vi "pick_and_place_sorting_weights_project.vi"() -> ()   [LabVIEW 2023]
uses:
  <vilib>/MakerHub/LINX/Public/Peripherals/Digital/Digital Write 1 Chan.vi
  <vilib>/MakerHub/LINX/Public/Peripherals/Digital/Digital Write N Chans.vi
  <vilib>/MakerHub/LINX/Private/Local IO/LinxDigitalWrite.vi
  <vilib>/MakerHub/LINX/Public/Utilities/Check Channel.vi
  <vilib>/MakerHub/LINX/Public/Utilities/Open Serial.vi
  <vilib>/MakerHub/LINX/Public/Sensors/Motion/Servo/Servo Open N Channels.vi
  <vilib>/Instr/_visa.llb/VISA Configure Serial Port (Instr).vi
  <vilib>/MakerHub/LINX/Private/Utilties/Generate Error.vi
  <vilib>/MakerHub/LINX/Public/Sensors/Motion/Servo/Servo Set Pulse Width N Channels.vi
  <vilib>/MakerHub/LINX/Public/Sensors/Motion/Servo/Servo Close N Channels.vi
  <vilib>/MakerHub/LINX/LMH-LINX.lvlib
  <vilib>/MakerHub/LINX/Public/Sensors/Motion/Servo/Servo.lvlib
panel:
  in  "load cell arduino serial port":refnum<visa-resource-name>="N/A"
  out "TO POS":i32[](array[numeric])
  out "FROM POS":i32[](array[numeric])
  out "CURRENT\nBOX POS":i32
  in  "main arduino serial port":refnum<visa-resource-name>="N/A"
  in  "lift servo\nchannel":u8 max=50 step=1
  in  "rotate servo\nchannel":u8 max=50 step=1
  in  "magnet\nchannel":u8 max=50 step=1
  in  "AUTO SORTING WEIGHTS":bool
  out "CONTROL MODE":bool
  in  "STOP PROGRAM":bool
  in  "BOXES POSITIONS":bool[](array[boolean])
  in  "LIFT":u32(slide) max=100 step=5 scale=0.0..100.0
  in  "MAGNET":bool caption="Boolean 2"
  out "BOXES WEIGHTS MEASUREMENTS":dbl[](array[numeric])
  out "CURRENT WEIGHT":dbl format="%#.1p"
  in  "ROTATE":u32(knob) caption="Up Button" max=260 step=5
  # "Pick and Place - Sorting Weights"
  # "Robotic arm control"
  # "Scale / weights control"
  # "1               2               3               4"
  # "o"
  # "%"
  # "gr"
  # "Initially, give the correct serial communication USB ports for the two arduinos and the right pins numbers to the servo, magnet and load cell channels, and then run the program. You can control the robotic arm manually (the joints' servomotors and the electromagent) using the controls of the \"Robotic arm control\" section. To start the \"auto sorting weights\" process, first you have to mark the positions of the boxes in the \"Scale / weights control\" section, before pressing the appropriate button."
  # "Boxes positions:\n1 -> 50 degrees\n2 -> 80 degrees\n3 -> 110 degrees\n4 -> 140 degrees\nScale position:\n5 -> 3 degrees"
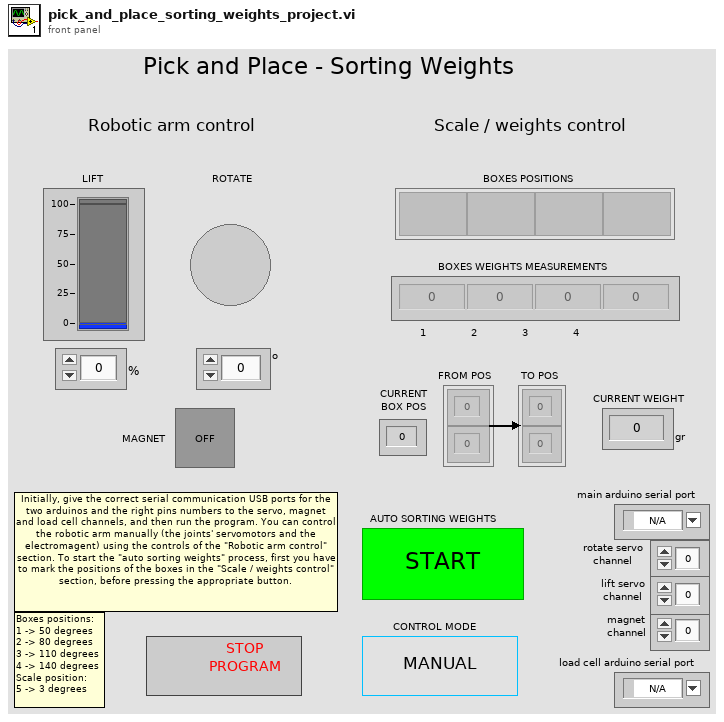
[diagram p1: front panel]
types:
  T1 = typedef "LMH-LINX.lvlib/LINX Ref.ctl" = cluster{"IO":T2, "Interface":T3, "LINX Device Config":T4}
  T2 = typedef "LMH-LINX.lvlib/Platform.ctl" = enum16{"Remote", "Local"}
  T3 = typedef "LMH-LINX.lvlib/Interface.ctl" = enum16{"Serial", "TCP"}
  T4 = typedef "LMH-LINX.lvlib/Device.lvlib/LINX Device Config.ctl" = cluster{"Interface":T3, "COM Port":refnum<visa-resource-name>, "TCP Configuration":T5, "Device Family":u8, "Device ID":u8, "Device Name":string, "TCP Ref":refnum<k5>, "Channels":T6}
  T5 = typedef "LMH-LINX.lvlib/Device.lvlib/TCP Config.ctl" = cluster{"IP Address":string, "Port":u16}
  T6 = typedef "LMH-LINX.lvlib/Channels.ctl" = cluster{"DI":u8[], "DO":u8[], "AI":u8[], "AO":u8[], "PWM":u8[], "QE":u8[], "UART":u8[], "I2C 2":u8[], "SPI":u8[], "CAN":u8[], "Servo":u8[], "AI Ref (V)":dbl, "AI Resolution (Bits)":u8, "AO Ref (V)":dbl, "AO Resolution (Bits)":u8}
  T7 = enum8{"Enabled", "Disabled", "Disabled and Grayed Out"}
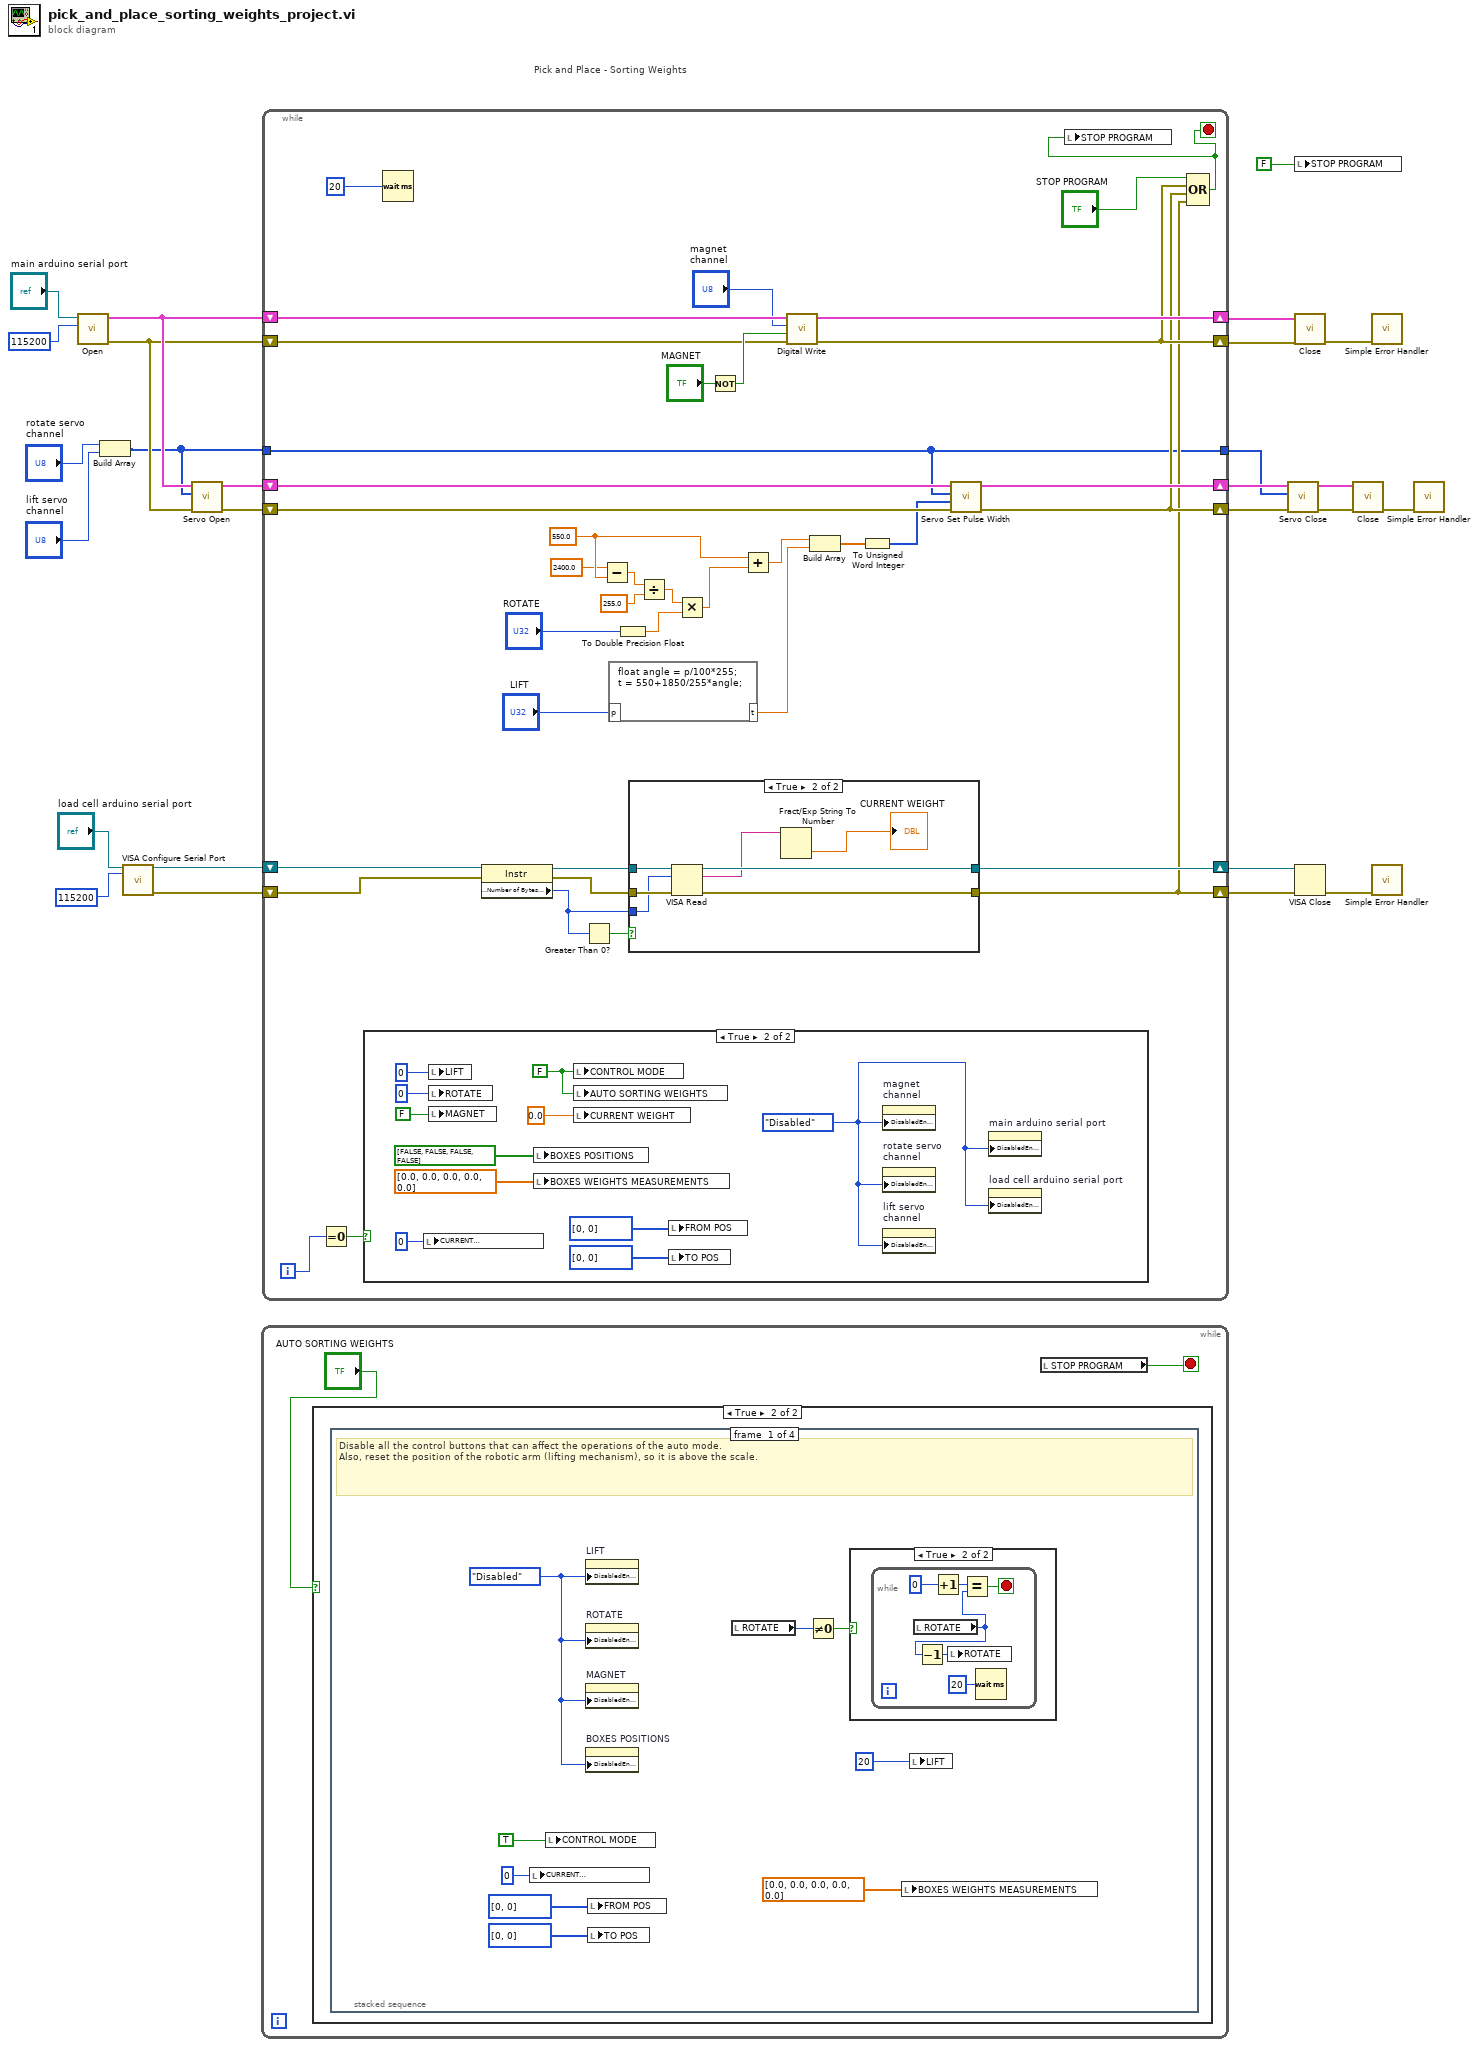
[diagram p0: block diagram]
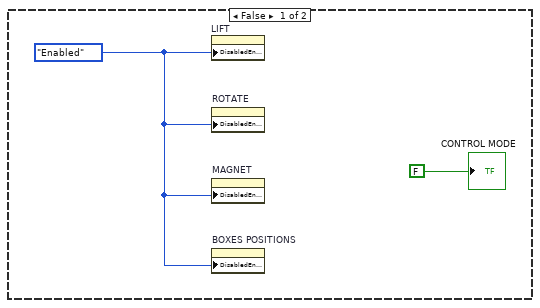
[diagram p2: hidden frame]
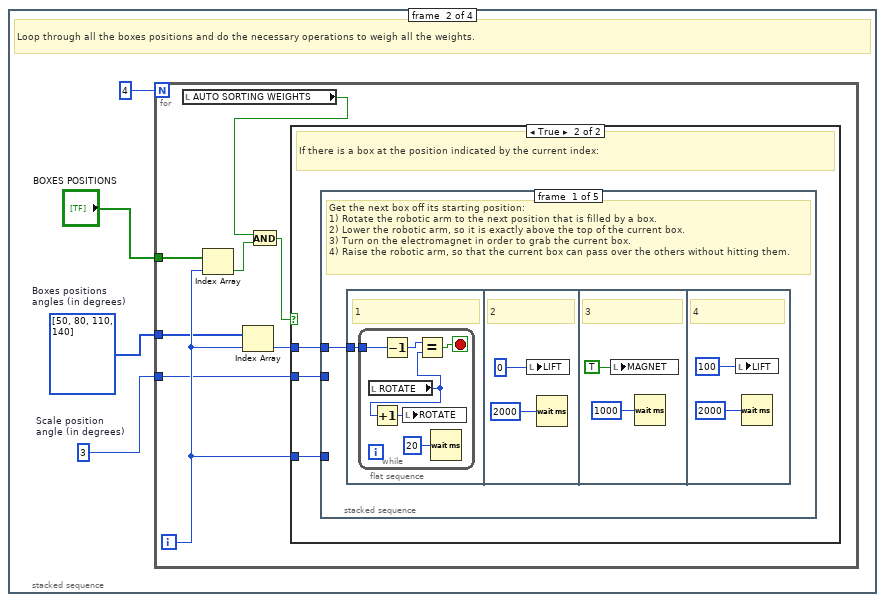
[diagram p4: hidden frame]
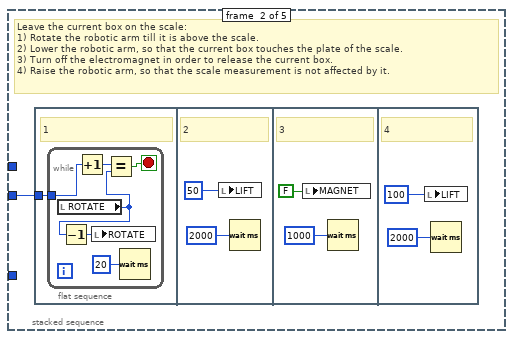
[diagram p6: hidden frame]
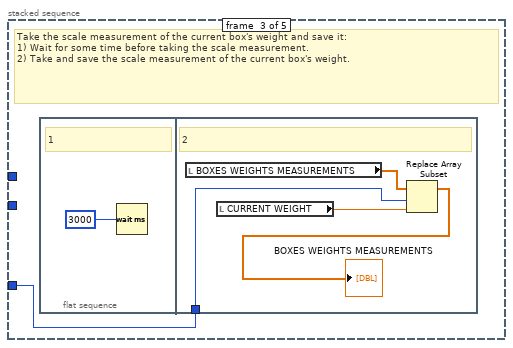
[diagram p7: hidden frame]
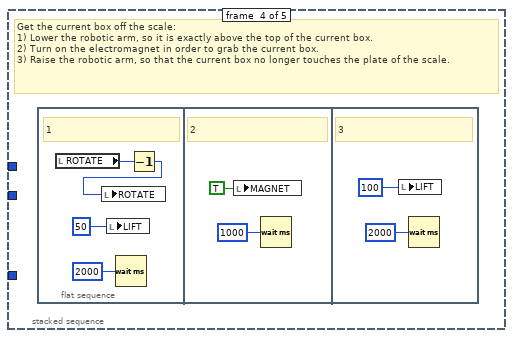
[diagram p8: hidden frame]
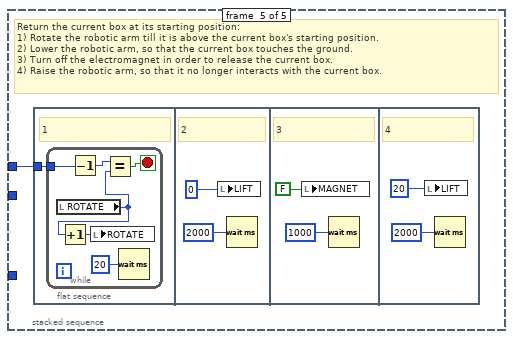
[diagram p9: hidden frame]
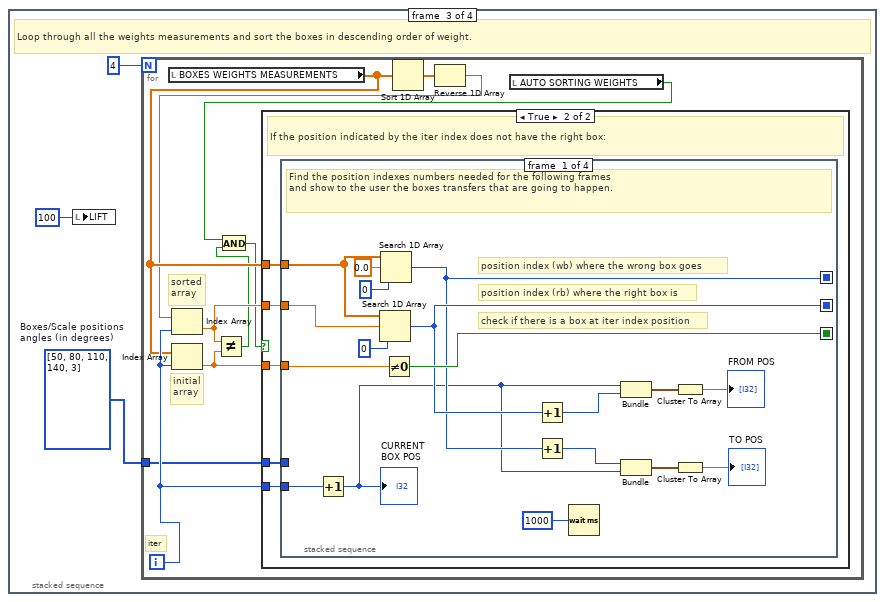
[diagram p10: hidden frame]
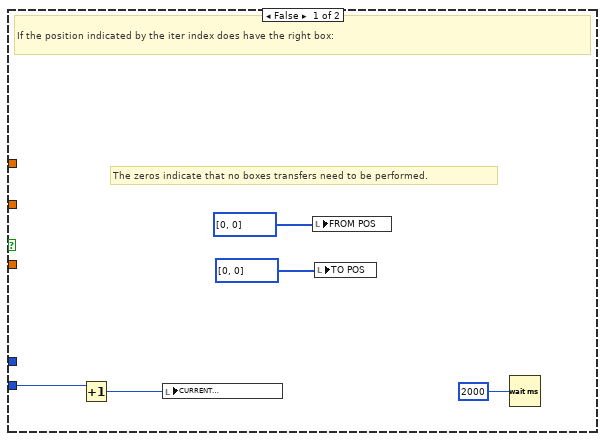
[diagram p11: hidden frame]
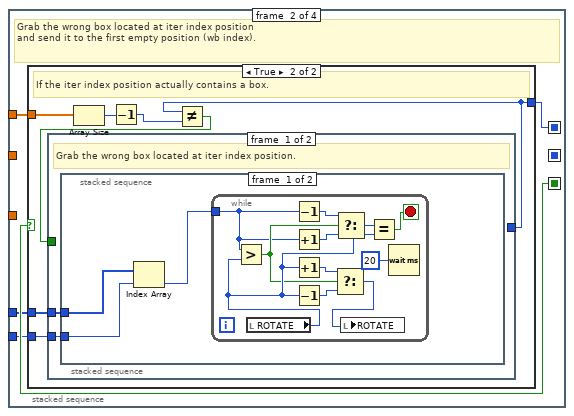
[diagram p12: hidden frame]
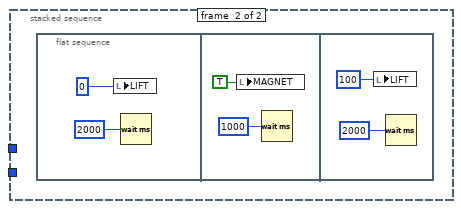
[diagram p14: hidden frame]
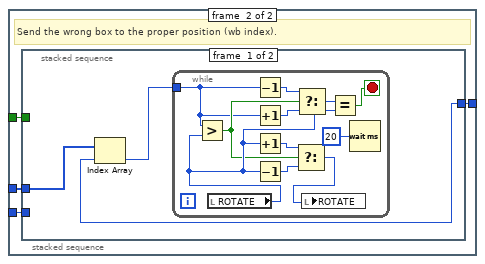
[diagram p15: hidden frame]
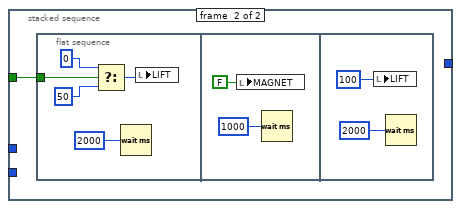
[diagram p16: hidden frame]
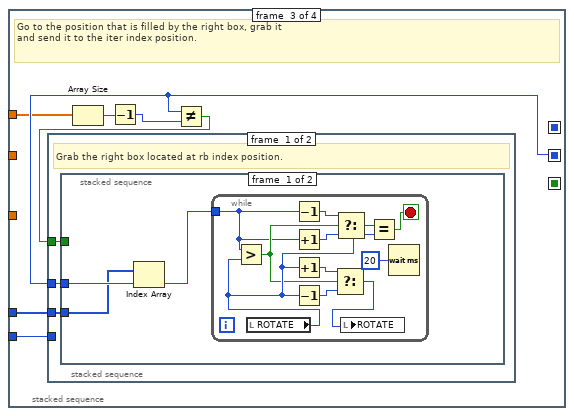
[diagram p17: hidden frame]
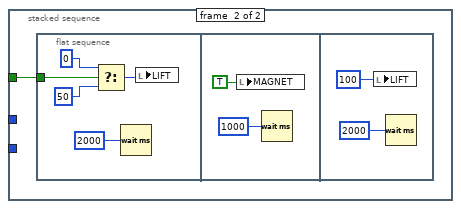
[diagram p18: hidden frame]
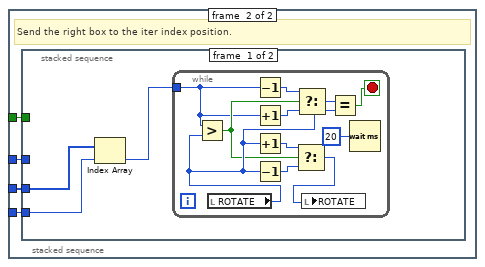
[diagram p19: hidden frame]
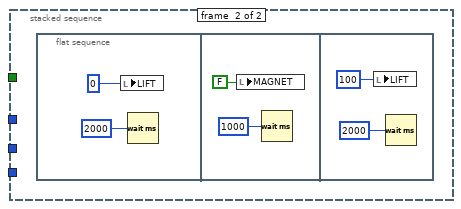
[diagram p20: hidden frame]
diagram:
  # "Pick and Place - Sorting Weights"
  n1 = call-poly <vilib>:"Open.vi"("Baud Rate Override"=u32 115200, "Serial Port"="main arduino serial port") -> ("Error Out"=w15:errorcluster, "LINX Resource"=w16:T1)  [unwired: 7 in, 1 out]
  n2 = Build Array("rotate servo\nchannel", "lift servo\nchannel") -> (w1:u8[])
  n3 = call-poly "VISA Configure Serial Port"("VISA resource name"="load cell arduino serial port", "baud rate (9600)"=u32 115200 ("baud rate (115200)")) -> ("VISA resource name out"=w10:refnum<visa-resource-name>, "error out"=w9:errorcluster)  [unwired: 12 in]
  n4 = call-poly <vilib>:"Servo Open.vi"("Error In"=w15, "Servo Channels"=w1, "LINX Resource"=w16) -> ("Error Out"=w18:errorcluster, "LINX Resource"=w20:T1)  [unwired: 7 in]
  n5 = while {
    stop <- w28 stop-if-true
    n6 = case shown="True" "AUTO SORTING WEIGHTS" {
      frame False {
        w29 = T7."Enabled" ("Disabled")
        n7 = property on="LIFT" class="Slide (strict)"("DisabledEnum"=w29) -> ()  [unwired: 2 in, 2 out]
        n8 = property on="ROTATE" class="Knob (strict)"("DisabledEnum"=w29) -> ()  [unwired: 2 in, 2 out]
        n9 = property on="MAGNET" class="Bool (strict)"("DisabledEnum"=w29) -> ()  [unwired: 2 in, 2 out]
        n10 = property on="BOXES POSITIONS" class="Arr (strict)"("DisabledEnum"=w29) -> ()  [unwired: 2 in, 2 out]
        "CONTROL MODE" <- FALSE ("CONTROL MODE")
      }
      frame True {
        n11 = stacked-sequence {
          frame #0 {
            w37 = T7."Disabled" ("Disabled")
            # "Disable all the control buttons that can affect the operations of the auto mode.\nAlso, reset the position of the robotic arm (lifting mechanism), so it is above the scale."
            n12 = local write "CURRENT\nBOX POS"(0 ("CURRENT\nBOX POS")) -> ()
            n13 = local write "CONTROL MODE"(TRUE ("CONTROL MODE")) -> ()
            n14 = property on="LIFT" class="Slide (strict)"("DisabledEnum"=w37) -> ()  [unwired: 2 in, 2 out]
            n15 = property on="ROTATE" class="Knob (strict)"("DisabledEnum"=w37) -> ()  [unwired: 2 in, 2 out]
            n16 = property on="MAGNET" class="Bool (strict)"("DisabledEnum"=w37) -> ()  [unwired: 2 in, 2 out]
            n17 = property on="BOXES POSITIONS" class="Arr (strict)"("DisabledEnum"=w37) -> ()  [unwired: 2 in, 2 out]
            n18 = local write "FROM POS"(i32[] [0, 0] ("FROM POS")) -> ()
            n19 = local write "TO POS"(i32[] [0, 0] ("TO POS")) -> ()
            n20 = local read "ROTATE"() -> (w32:u32)
            n21 = Not Equal To 0?(x=w32) -> (x != 0?=w33:bool)
            n22 = case shown="True" w33 {
              frame False {
              }
              frame True {
                n23 = while {
                  stop <- w43 stop-if-true
                  n24 = local read "ROTATE"() -> (w42:u32)
                  n25 = Decrement(x=w42) -> (x-1=w45:u32)
                  n26 = Increment(x=u32 0) -> (x+1=w41:u32)
                  n27 = local write "ROTATE"(w45) -> ()
                  n28 = Equal?(x=w41, y=w42) -> (x = y?=w43:bool)
                  n29 = Wait (ms)(milliseconds to wait=u32 20) -> ()  [unwired: 1 out]
                }
              }
            }
            n30 = local write "BOXES WEIGHTS MEASUREMENTS"(dbl[] [0.0, 0.0, 0.0, 0.0, 0.0] ("BOXES WEIGHTS MEASUREMENTS")) -> ()
            n31 = local write "LIFT"(u32 20 ("LIFT")) -> ()
          }
          frame #1 {
            w46 = u32 3  # Scale position angle (in degrees)
            w48 = u32[] [50, 80, 110, 140]  # Boxes positions angles (in degrees)
            # "Loop through all the boxes positions and do the necessary operations to weigh all the weights."
            n32 = for {
              N: 4 -> [_]
              tunnel: w48 -> [w55]
              tunnel: "BOXES POSITIONS" -> [w57]
              tunnel: w46 -> [w50]
              i -> [w56]
              n33 = local read "AUTO SORTING WEIGHTS"() -> (w53:bool)
              n34 = Index Array(array=w57, index=w56) -> (element=w51:bool)
              n35 = Index Array(array=w55, index=w56) -> (element=w54:u32)
              n36 = And(x=w53, y=w51) -> (x .and. y?=w52:bool)
              n37 = case shown="True" w52 {
                tunnel: w56 -> [_ w60]
                tunnel: w54 -> [_ w59]
                tunnel: w50 -> [_ w58]
                frame False {
                  # "No actions need to be performed in this case."
                  # "If the position indicated by the current index is empty:"
                }
                frame True {
                  # "If there is a box at the position indicated by the current index:"
                  n38 = stacked-sequence {
                    tunnel: w60 -> [_ _ w89 _ _]
                    tunnel: w59 -> [w61 _ _ _ w103]
                    tunnel: w58 -> [_ w75 _ _ _]
                    frame #0 {
                      # "Get the next box off its starting position:\n1) Rotate the robotic arm to the next position that is filled by a box.\n2) Lower the robotic arm, so it is exactly above the top of the current box.\n3) Turn on the electromagnet in order to grab the current box.\n4) Raise the robotic arm, so that the current box can pass over the others without hitting them."
                      n39 = flat-sequence {
                        tunnel: w61 -> [w62]
                        frame #0 {
                          # "1"
                          n40 = while {
                            tunnel: w62 -> [w63]
                            stop <- w66 stop-if-true
                            n41 = local read "ROTATE"() -> (w65:u32)
                            n42 = Increment(x=w65) -> (x+1=w68:u32)
                            n43 = Decrement(x=w63) -> (x-1=w64:u32)
                            n44 = local write "ROTATE"(w68) -> ()
                            n45 = Equal?(x=w64, y=w65) -> (x = y?=w66:bool)
                            n46 = Wait (ms)(milliseconds to wait=u32 20) -> ()  [unwired: 1 out]
                          }
                        }
                        frame #1 {
                          # "2"
                          n47 = local write "LIFT"(u32 0 ("LIFT")) -> ()
                          n48 = Wait (ms)(milliseconds to wait=u32 2000) -> ()  [unwired: 1 out]
                        }
                        frame #2 {
                          # "3"
                          n49 = local write "MAGNET"(TRUE ("MAGNET")) -> ()
                          n50 = Wait (ms)(milliseconds to wait=u32 1000) -> ()  [unwired: 1 out]
                        }
                        frame #3 {
                          # "4"
                          n51 = local write "LIFT"(u32 100 ("LIFT")) -> ()
                          n52 = Wait (ms)(milliseconds to wait=u32 2000) -> ()  [unwired: 1 out]
                        }
                      }
                    }
                    frame #1 {
                      # "Leave the current box on the scale:\n1) Rotate the robotic arm till it is above the scale.\n2) Lower the robotic arm, so that the current box touches the plate of the scale.\n3) Turn off the electromagnet in order to release the current box.\n4) Raise the robotic arm, so that the scale measurement is not affected by it."
                      n53 = flat-sequence {
                        tunnel: w75 -> [w76]
                        frame #0 {
                          # "1"
                          n54 = while {
                            tunnel: w76 -> [w78]
                            stop <- w80 stop-if-true
                            n55 = local read "ROTATE"() -> (w79:u32)
                            n56 = Decrement(x=w79) -> (x-1=w82:u32)
                            n57 = Increment(x=w78) -> (x+1=w77:u32)
                            n58 = local write "ROTATE"(w82) -> ()
                            n59 = Equal?(x=w77, y=w79) -> (x = y?=w80:bool)
                            n60 = Wait (ms)(milliseconds to wait=u32 20) -> ()  [unwired: 1 out]
                          }
                        }
                        frame #1 {
                          # "2"
                          n61 = local write "LIFT"(u32 50 ("LIFT")) -> ()
                          n62 = Wait (ms)(milliseconds to wait=u32 2000) -> ()  [unwired: 1 out]
                        }
                        frame #2 {
                          # "3"
                          n63 = local write "MAGNET"(FALSE ("MAGNET")) -> ()
                          n64 = Wait (ms)(milliseconds to wait=u32 1000) -> ()  [unwired: 1 out]
                        }
                        frame #3 {
                          # "4"
                          n65 = local write "LIFT"(u32 100 ("LIFT")) -> ()
                          n66 = Wait (ms)(milliseconds to wait=u32 2000) -> ()  [unwired: 1 out]
                        }
                      }
                    }
                    frame #2 {
                      # "Take the scale measurement of the current box's weight and save it:\n1) Wait for some time before taking the scale measurement.\n2) Take and save the scale measurement of the current box's weight."
                      n67 = flat-sequence {
                        tunnel: w89 -> [w93]
                        frame #0 {
                          # "1"
                          n68 = Wait (ms)(milliseconds to wait=u32 3000) -> ()  [unwired: 1 out]
                        }
                        frame #1 {
                          # "2"
                          n69 = local read "BOXES WEIGHTS MEASUREMENTS"() -> (w94:dbl[])
                          n70 = local read "CURRENT WEIGHT"() -> (w92:dbl)
                          n71 = Replace Array Subset(array=w94, new element=w92, index=w93) -> (→"BOXES WEIGHTS MEASUREMENTS":dbl[])
                        }
                      }
                    }
                    frame #3 {
                      # "Get the current box off the scale:\n1) Lower the robotic arm, so it is exactly above the top of the current box.\n2) Turn on the electromagnet in order to grab the current box.\n3) Raise the robotic arm, so that the current box no longer touches the plate of the scale."
                      n72 = flat-sequence {
                        frame #0 {
                          # "1"
                          n73 = local read "ROTATE"() -> (w96:u32)
                          n74 = local write "LIFT"(u32 50 ("LIFT")) -> ()
                          n75 = Wait (ms)(milliseconds to wait=u32 2000) -> ()  [unwired: 1 out]
                          n76 = Decrement(x=w96) -> (x-1=w95:u32)
                          n77 = local write "ROTATE"(w95) -> ()
                        }
                        frame #1 {
                          # "2"
                          n78 = local write "MAGNET"(TRUE ("MAGNET")) -> ()
                          n79 = Wait (ms)(milliseconds to wait=u32 1000) -> ()  [unwired: 1 out]
                        }
                        frame #2 {
                          # "3"
                          n80 = local write "LIFT"(u32 100 ("LIFT")) -> ()
                          n81 = Wait (ms)(milliseconds to wait=u32 2000) -> ()  [unwired: 1 out]
                        }
                      }
                    }
                    frame #4 {
                      # "Return the current box at its starting position:\n1) Rotate the robotic arm till it is above the current box's starting position.\n2) Lower the robotic arm, so that the current box touches the ground.\n3) Turn off the electromagnet in order to release the current box.\n4) Raise the robotic arm, so that it no longer interacts with the current box."
                      n82 = flat-sequence {
                        tunnel: w103 -> [w104]
                        frame #0 {
                          # "1"
                          n83 = while {
                            tunnel: w104 -> [w106]
                            stop <- w108 stop-if-true
                            n84 = local read "ROTATE"() -> (w107:u32)
                            n85 = Increment(x=w107) -> (x+1=w110:u32)
                            n86 = Decrement(x=w106) -> (x-1=w105:u32)
                            n87 = local write "ROTATE"(w110) -> ()
                            n88 = Equal?(x=w105, y=w107) -> (x = y?=w108:bool)
                            n89 = Wait (ms)(milliseconds to wait=u32 20) -> ()  [unwired: 1 out]
                          }
                        }
                        frame #1 {
                          # "2"
                          n90 = local write "LIFT"(u32 0 ("LIFT")) -> ()
                          n91 = Wait (ms)(milliseconds to wait=u32 2000) -> ()  [unwired: 1 out]
                        }
                        frame #2 {
                          # "3"
                          n92 = local write "MAGNET"(FALSE ("MAGNET")) -> ()
                          n93 = Wait (ms)(milliseconds to wait=u32 1000) -> ()  [unwired: 1 out]
                        }
                        frame #3 {
                          # "4"
                          n94 = local write "LIFT"(u32 20 ("LIFT")) -> ()
                          n95 = Wait (ms)(milliseconds to wait=u32 2000) -> ()  [unwired: 1 out]
                        }
                      }
                    }
                  }
                }
              }
            }
          }
          frame #2 {
            w118 = u32[] [50, 80, 110, 140, 3]  # Boxes/Scale positions angles (in degrees)
            # "Loop through all the weights measurements and sort the boxes in descending order of weight."
            n96 = local write "LIFT"(u32 100 ("LIFT")) -> ()
            n97 = for {
              N: 4 -> [_]
              tunnel: w118 -> [w126]
              i -> [w127]
              # "iter"
              # "initial\narray"
              # "sorted\narray"
              n98 = local read "BOXES WEIGHTS MEASUREMENTS"() -> (w124:dbl[])
              n99 = Index Array(array=w124, index=w127) -> (element=w128:dbl)
              n100 = Sort 1D Array(array=w124) -> (sorted array=w125:dbl[])
              n101 = Reverse 1D Array(array=w125) -> (reversed array=w123:dbl[])
              n102 = Index Array(array=w123, index=w127) -> (element=w129:dbl)
              n103 = Not Equal?(x=w129, y=w128) -> (x != y?=w121:bool)
              n104 = local read "AUTO SORTING WEIGHTS"() -> (w122:bool)
              n105 = And(x=w122, y=w121) -> (x .and. y?=w120:bool)
              n106 = case shown="True" w120 {
                tunnel: w129 -> [_ w138]
                tunnel: w128 -> [_ w139]
                tunnel: w124 -> [_ w137]
                tunnel: w127 -> [w134 w136]
                tunnel: w126 -> [_ w135]
                frame False {
                  # "The zeros indicate that no boxes transfers need to be performed."
                  # "If the position indicated by the iter index does have the right box:"
                  n107 = Increment(x=w134) -> (x+1=w133:i32)
                  n108 = local write "CURRENT\nBOX POS"(w133) -> ()
                  n109 = local write "FROM POS"(i32[] [0, 0] ("FROM POS")) -> ()
                  n110 = local write "TO POS"(i32[] [0, 0] ("TO POS")) -> ()
                  n111 = Wait (ms)(milliseconds to wait=u32 2000) -> ()  [unwired: 1 out]
                }
                frame True {
                  # "If the position indicated by the iter index does not have the right box:"
                  n112 = stacked-sequence {
                    seq-local: [w142 _ _ _] -> [_ w160 _ w282]
                    seq-local: [w148 _ _ _] -> [_ _ w226 w278]
                    seq-local: [w154 _ _ _] -> [_ w162 _ _]
                    tunnel: w139 -> [w151 _ _ w281]
                    tunnel: w138 -> [w152 _ _ w279]
                    tunnel: w137 -> [w153 w161 w225 w283]
                    tunnel: w136 -> [w150 w159 w224 w280]
                    tunnel: w135 -> [_ w158 w220 _]
                    frame #0 {
                      # "check if there is a box at iter index position"
                      # "position index (rb) where the right box is"
                      # "position index (wb) where the wrong box goes"
                      # "Find the position indexes numbers needed for the following frames\nand show to the user the boxes transfers that are going to happen."
                      n113 = Increment(x=w150) -> (x+1=w141:i32)
                      "CURRENT\nBOX POS" <- w141
                      n114 = Search 1D Array(1D array=w153, element=w152, start index (0)=0) -> (index of element=w148:i32)
                      n115 = Search 1D Array(1D array=w153, element=0.0, start index (0)=0) -> (index of element=w142:i32)
                      n116 = Not Equal To 0?(x=w151) -> (x != 0?=w154:bool)
                      n117 = Increment(x=w148) -> (x+1=w147:i32)
                      n118 = Increment(x=w142) -> (x+1=w143:i32)
                      n119 = Wait (ms)(milliseconds to wait=u32 1000) -> ()  [unwired: 1 out]
                      n120 = Bundle(w141, w147) -> (w146:cluster{i32, i32})  [unwired: 1 in]
                      n121 = Bundle(w143, w141) -> (w145:cluster{i32, i32})  [unwired: 1 in]
                      n122 = Cluster To Array(cluster=w146) -> (array=→"FROM POS":i32[])
                      n123 = Cluster To Array(cluster=w145) -> (array=→"TO POS":i32[])
                    }
                    frame #1 {
                      # "Grab the wrong box located at iter index position\nand send it to the first empty position (wb index)."
                      n124 = case shown="True" w162 {
                        tunnel: w161 -> [_ w169]
                        tunnel: w160 -> [_ w164]
                        tunnel: w159 -> [_ w165]
                        tunnel: w158 -> [_ w163]
                        frame False {
                          # "No actions need to be performed in this case."
                          # "If the iter index position does not contain a box."
                        }
                        frame True {
                          # "If the iter index position actually contains a box."
                          n125 = Array Size(array=w169) -> (size(s)=w168:i32)
                          n126 = Decrement(x=w168) -> (x-1=w167:i32)
                          n127 = Not Equal?(x=w164, y=w167) -> (x != y?=w166:bool)
                          n128 = stacked-sequence {
                            tunnel: w166 -> [_ w195]
                            tunnel: w165 -> [w171 w194]
                            tunnel: w164 -> [_ w193]
                            tunnel: w163 -> [w170 w192]
                            frame #0 {
                              # "Grab the wrong box located at iter index position."
                              n129 = stacked-sequence {
                                tunnel: w171 -> [w173 _]
                                tunnel: w170 -> [w172 _]
                                frame #0 {
                                n130 = Index Array(array=w172, index=w173) -> (element=w174:u32)
                                n131 = while {
                                tunnel: w174 -> [w176]
                                tunnel: [w176] -> _
                                stop <- w185 stop-if-true
                                n132 = local read "ROTATE"() -> (w178:u32)
                                n133 = Greater?(x=w176, y=w178) -> (0:w177:bool)
                                n134 = Decrement(x=w176) -> (x-1=w180:u32)
                                n135 = Increment(x=w176) -> (x+1=w181:u32)
                                n136 = Increment(x=w178) -> (x+1=w183:u32)
                                n137 = Decrement(x=w178) -> (x-1=w182:u32)
                                n138 = Select(t=w183, s=w177, f=w182) -> (s? t:f=w184:u32)
                                n139 = Select(t=w180, s=w177, f=w181) -> (s? t:f=w179:u32)
                                n140 = local write "ROTATE"(w184) -> ()
                                n141 = Equal?(x=w179, y=w178) -> (x = y?=w185:bool)
                                n142 = Wait (ms)(milliseconds to wait=u32 20) -> ()  [unwired: 1 out]
                                }
                                }
                                frame #1 {
                                n143 = flat-sequence {
                                frame #0 {
                                n144 = local write "LIFT"(u32 0 ("LIFT")) -> ()
                                n145 = Wait (ms)(milliseconds to wait=u32 2000) -> ()  [unwired: 1 out]
                                }
                                frame #1 {
                                n146 = local write "MAGNET"(TRUE ("MAGNET")) -> ()
                                n147 = Wait (ms)(milliseconds to wait=u32 1000) -> ()  [unwired: 1 out]
                                }
                                frame #2 {
                                n148 = local write "LIFT"(u32 100 ("LIFT")) -> ()
                                n149 = Wait (ms)(milliseconds to wait=u32 2000) -> ()  [unwired: 1 out]
                                }
                                }
                                }
                              }
                            }
                            frame #1 {
                              # "Send the wrong box to the proper position (wb index)."
                              n150 = stacked-sequence {
                                tunnel: w195 -> [_ w210]
                                tunnel: w194 -> [_ _]
                                tunnel: w193 -> [w197 _]
                                tunnel: w192 -> [w196 _]
                                frame #0 {
                                n151 = Index Array(array=w196, index=w197) -> (element=w198:u32)
                                n152 = while {
                                tunnel: w198 -> [w200]
                                tunnel: [w200] -> _
                                stop <- w209 stop-if-true
                                n153 = local read "ROTATE"() -> (w202:u32)
                                n154 = Greater?(x=w200, y=w202) -> (0:w201:bool)
                                n155 = Decrement(x=w200) -> (x-1=w204:u32)
                                n156 = Increment(x=w200) -> (x+1=w205:u32)
                                n157 = Increment(x=w202) -> (x+1=w207:u32)
                                n158 = Decrement(x=w202) -> (x-1=w206:u32)
                                n159 = Select(t=w207, s=w201, f=w206) -> (s? t:f=w208:u32)
                                n160 = Select(t=w204, s=w201, f=w205) -> (s? t:f=w203:u32)
                                n161 = local write "ROTATE"(w208) -> ()
                                n162 = Equal?(x=w203, y=w202) -> (x = y?=w209:bool)
                                n163 = Wait (ms)(milliseconds to wait=u32 20) -> ()  [unwired: 1 out]
                                }
                                }
                                frame #1 {
                                n164 = flat-sequence {
                                tunnel: w210 -> [w211]
                                frame #0 {
                                n165 = Select(t=u32 0, s=w211, f=u32 50) -> (s? t:f=w215:u32)
                                n166 = Wait (ms)(milliseconds to wait=u32 2000) -> ()  [unwired: 1 out]
                                n167 = local write "LIFT"(w215) -> ()
                                }
                                frame #1 {
                                n168 = local write "MAGNET"(FALSE ("MAGNET")) -> ()
                                n169 = Wait (ms)(milliseconds to wait=u32 1000) -> ()  [unwired: 1 out]
                                }
                                frame #2 {
                                n170 = local write "LIFT"(u32 100 ("LIFT")) -> ()
                                n171 = Wait (ms)(milliseconds to wait=u32 2000) -> ()  [unwired: 1 out]
                                }
                                }
                                }
                              }
                            }
                          }
                        }
                      }
                    }
                    frame #2 {
                      # "Go to the position that is filled by the right box, grab it\nand send it to the iter index position."
                      n172 = Array Size(array=w225) -> (size(s)=w222:i32)
                      n173 = Decrement(x=w222) -> (x-1=w223:i32)
                      n174 = Not Equal?(x=w226, y=w223) -> (x != y?=w221:bool)
                      n175 = stacked-sequence {
                        tunnel: w221 -> [w229 w257]
                        tunnel: w226 -> [w228 w256]
                        tunnel: w224 -> [_ w255]
                        tunnel: w220 -> [w227 w254]
                        frame #0 {
                          # "Grab the right box located at rb index position."
                          n176 = stacked-sequence {
                            tunnel: w229 -> [_ w244]
                            tunnel: w228 -> [w231 _]
                            tunnel: w227 -> [w230 _]
                            frame #0 {
                              n177 = Index Array(array=w230, index=w231) -> (element=w232:u32)
                              n178 = while {
                                tunnel: w232 -> [w234]
                                tunnel: [w234] -> _
                                stop <- w243 stop-if-true
                                n179 = local read "ROTATE"() -> (w236:u32)
                                n180 = Greater?(x=w234, y=w236) -> (0:w235:bool)
                                n181 = Decrement(x=w234) -> (x-1=w238:u32)
                                n182 = Increment(x=w234) -> (x+1=w239:u32)
                                n183 = Increment(x=w236) -> (x+1=w241:u32)
                                n184 = Decrement(x=w236) -> (x-1=w240:u32)
                                n185 = Select(t=w241, s=w235, f=w240) -> (s? t:f=w242:u32)
                                n186 = Select(t=w238, s=w235, f=w239) -> (s? t:f=w237:u32)
                                n187 = local write "ROTATE"(w242) -> ()
                                n188 = Equal?(x=w237, y=w236) -> (x = y?=w243:bool)
                                n189 = Wait (ms)(milliseconds to wait=u32 20) -> ()  [unwired: 1 out]
                              }
                            }
                            frame #1 {
                              n190 = flat-sequence {
                                tunnel: w244 -> [w245]
                                frame #0 {
                                n191 = Select(t=u32 0, s=w245, f=u32 50) -> (s? t:f=w249:u32)
                                n192 = Wait (ms)(milliseconds to wait=u32 2000) -> ()  [unwired: 1 out]
                                n193 = local write "LIFT"(w249) -> ()
                                }
                                frame #1 {
                                n194 = local write "MAGNET"(TRUE ("MAGNET")) -> ()
                                n195 = Wait (ms)(milliseconds to wait=u32 1000) -> ()  [unwired: 1 out]
                                }
                                frame #2 {
                                n196 = local write "LIFT"(u32 100 ("LIFT")) -> ()
                                n197 = Wait (ms)(milliseconds to wait=u32 2000) -> ()  [unwired: 1 out]
                                }
                              }
                            }
                          }
                        }
                        frame #1 {
                          # "Send the right box to the iter index position."
                          n198 = stacked-sequence {
                            tunnel: w257 -> [_ _]
                            tunnel: w256 -> [_ _]
                            tunnel: w255 -> [w259 _]
                            tunnel: w254 -> [w258 _]
                            frame #0 {
                              n199 = Index Array(array=w258, index=w259) -> (element=w260:u32)
                              n200 = while {
                                tunnel: w260 -> [w262]
                                tunnel: [w262] -> _
                                stop <- w271 stop-if-true
                                n201 = local read "ROTATE"() -> (w264:u32)
                                n202 = Greater?(x=w262, y=w264) -> (0:w263:bool)
                                n203 = Decrement(x=w262) -> (x-1=w266:u32)
                                n204 = Increment(x=w262) -> (x+1=w267:u32)
                                n205 = Increment(x=w264) -> (x+1=w269:u32)
                                n206 = Decrement(x=w264) -> (x-1=w268:u32)
                                n207 = Select(t=w269, s=w263, f=w268) -> (s? t:f=w270:u32)
                                n208 = Select(t=w266, s=w263, f=w267) -> (s? t:f=w265:u32)
                                n209 = local write "ROTATE"(w270) -> ()
                                n210 = Equal?(x=w265, y=w264) -> (x = y?=w271:bool)
                                n211 = Wait (ms)(milliseconds to wait=u32 20) -> ()  [unwired: 1 out]
                              }
                            }
                            frame #1 {
                              n212 = flat-sequence {
                                frame #0 {
                                n213 = local write "LIFT"(u32 0 ("LIFT")) -> ()
                                n214 = Wait (ms)(milliseconds to wait=u32 2000) -> ()  [unwired: 1 out]
                                }
                                frame #1 {
                                n215 = local write "MAGNET"(FALSE ("MAGNET")) -> ()
                                n216 = Wait (ms)(milliseconds to wait=u32 1000) -> ()  [unwired: 1 out]
                                }
                                frame #2 {
                                n217 = local write "LIFT"(u32 100 ("LIFT")) -> ()
                                n218 = Wait (ms)(milliseconds to wait=u32 2000) -> ()  [unwired: 1 out]
                                }
                              }
                            }
                          }
                        }
                      }
                    }
                    frame #3 {
                      # "Update the \"BOXES WEIGHTS MEASUREMENTS\" array based on \nthe changes that occured in this iteration."
                      n219 = Replace Array Subset(array=w283, new element=w281, index=w282) -> (w284:dbl[])
                      n220 = Replace Array Subset(array=w284, new element=0.0 ("new element/subarray"), index=w278) -> (w286:dbl[])
                      n221 = Replace Array Subset(array=w286, new element=w279, index=w280) -> (w287:dbl[])
                      n222 = local write "BOXES WEIGHTS MEASUREMENTS"(w284) -> ()
                      n223 = local write "BOXES WEIGHTS MEASUREMENTS"(w286) -> ()
                      n224 = local write "BOXES WEIGHTS MEASUREMENTS"(w287) -> ()
                    }
                  }
                }
              }
            }
          }
          frame #3 {
            w289 = T7."Enabled" ("Disabled")
            # "The boxes have been sorted. Send a suitable message to the user.\nAlso, reset the position of the robotic arm (lifting mechanism), so it is above the scale."
            n225 = local write "CURRENT\nBOX POS"(0 ("CURRENT\nBOX POS")) -> ()
            n226 = local write "CONTROL MODE"(FALSE ("CONTROL MODE")) -> ()
            n227 = property on="LIFT" class="Slide (strict)"("DisabledEnum"=w289) -> ()  [unwired: 2 in, 2 out]
            n228 = property on="ROTATE" class="Knob (strict)"("DisabledEnum"=w289) -> ()  [unwired: 2 in, 2 out]
            n229 = property on="MAGNET" class="Bool (strict)"("DisabledEnum"=w289) -> ()  [unwired: 2 in, 2 out]
            n230 = property on="BOXES POSITIONS" class="Arr (strict)"("DisabledEnum"=w289) -> ()  [unwired: 2 in, 2 out]
            n231 = local write "FROM POS"(i32[] [0, 0] ("FROM POS")) -> ()
            n232 = local write "TO POS"(i32[] [0, 0] ("TO POS")) -> ()
            n233 = local read "ROTATE"() -> (w294:u32)
            n234 = Not Equal To 0?(x=w294) -> (x != 0?=w295:bool)
            n235 = case shown="True" w295 {
              frame False {
              }
              frame True {
                n236 = while {
                  stop <- w302 stop-if-true
                  n237 = local read "ROTATE"() -> (w301:u32)
                  n238 = Decrement(x=w301) -> (x-1=w304:u32)
                  n239 = Increment(x=u32 0) -> (x+1=w300:u32)
                  n240 = local write "ROTATE"(w304) -> ()
                  n241 = Equal?(x=w300, y=w301) -> (x = y?=w302:bool)
                  n242 = Wait (ms)(milliseconds to wait=u32 20) -> ()  [unwired: 1 out]
                }
              }
            }
            n243 = local write "AUTO SORTING WEIGHTS"(FALSE ("AUTO SORTING WEIGHTS")) -> ()
            n244 = local write "LIFT"(u32 20 ("LIFT")) -> ()
            n245 = One Button Dialog(message="The boxes have been sorted in\ndescending order of weight!", button name ("OK")="OK") -> ()  [unwired: 1 out]
          }
        }
      }
    }
    n246 = local read "STOP PROGRAM"() -> (w28:bool)
  }
  n247 = while {
    shift-right: [w341] -> w25
    shift-left: w16 -> [w338]
    shift-right: [w331] -> w24
    shift-left: w15 -> [w339]
    shift-right: [w336] -> w19
    shift-left: w20 -> [w337]
    shift-right: [w330] -> w17
    shift-left: w18 -> [w335]
    tunnel: [w305] -> w2
    tunnel: w1 -> [w305]
    shift-right: [w314] -> w7
    shift-left: w10 -> [w316]
    shift-right: [w312] -> w6
    shift-left: w9 -> [w315]
    i -> [w334]
    stop <- w310 stop-if-true
    w322 = 550.0 ("x")
    n248 = Equal To 0?(x=w334) -> (x = 0?=w333:bool)
    n249 = case shown="True" w333 {
      frame False {
      }
      frame True {
        w352 = T7."Disabled" ("Disabled")
        w356 = FALSE ("CONTROL MODE")
        n250 = local write "CURRENT\nBOX POS"(0 ("CURRENT\nBOX POS")) -> ()
        n251 = local write "LIFT"(u32 0 ("LIFT")) -> ()
        n252 = local write "ROTATE"(u32 0 ("ROTATE")) -> ()
        n253 = local write "MAGNET"(FALSE ("MAGNET")) -> ()
        n254 = local write "BOXES POSITIONS"(bool[] [FALSE, FALSE, FALSE, FALSE] ("BOXES POSITIONS")) -> ()
        n255 = local write "BOXES WEIGHTS MEASUREMENTS"(dbl[] [0.0, 0.0, 0.0, 0.0, 0.0] ("BOXES WEIGHTS MEASUREMENTS")) -> ()
        n256 = local write "CONTROL MODE"(w356) -> ()
        n257 = local write "AUTO SORTING WEIGHTS"(w356) -> ()
        n258 = local write "CURRENT WEIGHT"(0.0 ("CURRENT WEIGHT")) -> ()
        n259 = local write "FROM POS"(i32[] [0, 0] ("FROM POS")) -> ()
        n260 = local write "TO POS"(i32[] [0, 0] ("TO POS")) -> ()
        n261 = property on="magnet\nchannel" class="DigNum (strict)"("DisabledEnum"=w352) -> ()  [unwired: 2 in, 2 out]
        n262 = property on="rotate servo\nchannel" class="DigNum (strict)"("DisabledEnum"=w352) -> ()  [unwired: 2 in, 2 out]
        n263 = property on="lift servo\nchannel" class="DigNum (strict)"("DisabledEnum"=w352) -> ()  [unwired: 2 in, 2 out]
        n264 = property on="main arduino serial port" class="VISAName"("DisabledEnum"=w352) -> ()  [unwired: 2 in, 2 out]
        n265 = property on="load cell arduino serial port" class="VISAName"("DisabledEnum"=w352) -> ()  [unwired: 2 in, 2 out]
      }
    }
    n266 = Wait (ms)(milliseconds to wait=u32 20) -> ()  [unwired: 1 out]
    n267 = property class="Instr"(reference=w316, error in=w315) -> (reference out=w319:refnum<visa-resource-name>, error out=w318:errorcluster, "Serial Settings:Number of Bytes at Serial Port"=w313:u32)
    n268 = Greater Than 0?(x=w313) -> (x > 0?=w317:bool)
    n269 = Subtract(x=2400.0, y=w322) -> (x-y=w324:dbl)
    n270 = formula code="float angle = p/100*255;\nt = 550+1850/255*angle;"("p"="LIFT") -> ("t"=w307:dbl)
    n271 = To Double Precision Float(number="ROTATE") -> (double precision float=w323:dbl)
    n272 = case shown="True" w317 {
      tunnel: [w343 w351] -> w312
      tunnel: [w344 w350] -> w314
      tunnel: w319 -> [w344 w348]
      tunnel: w318 -> [w343 w347]
      tunnel: w313 -> [_ w346]
      frame False {
      }
      frame True {
        n273 = VISA Read(VISA resource name=w348, byte count=w346, error in (no error)=w347) -> (VISA resource name out=w350:refnum<visa-resource-name>, read buffer=w349:string, error out=w351:errorcluster)  [unwired: 1 out]
        n274 = Fract/Exp String To Number(string=w349) -> (number=→"CURRENT WEIGHT":dbl)  [unwired: 3 in, 1 out]
      }
    }
    n275 = Divide(x=w324, y=255.0) -> (x/y=w325:dbl)
    n276 = Multiply(x=w325, y=w323) -> (x*y=w326:dbl)
    n277 = Not(x="MAGNET") -> (.not. x?=w342:bool)
    n278 = Add(x=w322, y=w326) -> (x+y=w308:dbl)
    n279 = call-poly <vilib>:"Digital Write.vi"("Error In"=w339, "Output Value"=w342, "DO Channel"="magnet\nchannel", "LINX Resource"=w338) -> ("Error Out"=w331:errorcluster, "LINX Resource"=w341:T1)  [unwired: 6 in]
    n280 = Build Array(w308, w307) -> (w306:dbl[])
    n281 = To Unsigned Word Integer(number=w306) -> (unsigned 16bit integer=w309:u16[])
    n282 = call-poly <vilib>:"Servo Set Pulse Width.vi"("Error In"=w335, "Pulse Widths (uS)"=w309, "Servo Channels"=w305, "LINX Resource"=w337) -> ("Error Out"=w330:errorcluster, "LINX Resource"=w336:T1)  [unwired: 6 in]
    n283 = Compound Arithmetic op=OR("STOP PROGRAM", w331, w330, w312) -> (w310:bool)
    n284 = local write "STOP PROGRAM"(w310) -> ()
  }
  n285 = call-poly <vilib>:"Servo Close.vi"("Error In"=w17, "Servo Channels"=w2, "LINX Resource"=w19) -> ("Error Out"=w23:errorcluster, "LINX Resource"=w22:T1)  [unwired: 7 in]
  n286 = local write "STOP PROGRAM"(FALSE ("STOP PROGRAM")) -> ()
  n287 = call <vilib>:"Close.vi"("Error In"=w24, "LINX Resource"=w25) -> ("Error Out"=w26:errorcluster)  [unwired: 9 in]
  n288 = VISA Close(VISA resource name=w7, error in (no error)=w6) -> (error out=w8:errorcluster)
  n289 = call <vilib>:"Close.vi"("Error In"=w23, "LINX Resource"=w22) -> ("Error Out"=w21:errorcluster)  [unwired: 9 in]
  n290 = call <vilib>:"Simple Error Handler.vi"("error in (no error)"=w26) -> ()  [unwired: 4 in, 5 out]
  n291 = call <vilib>:"Simple Error Handler.vi"("error in (no error)"=w8) -> ()  [unwired: 4 in, 5 out]
  n292 = call <vilib>:"Simple Error Handler.vi"("error in (no error)"=w21) -> ()  [unwired: 4 in, 5 out]
